vi "testFIFO.vi"() -> ()   [LabVIEW 2019]
panel:
  out "output array":dbl[](array[numeric])
  in  "Stop 2":bool
  out "average":dbl
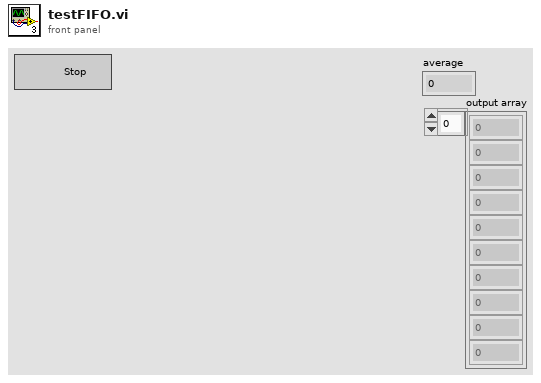
[diagram p1: front panel]
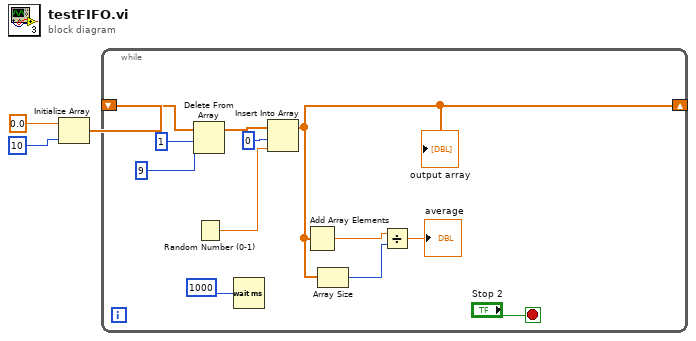
[diagram p0: block diagram]
diagram:
  n1 = Initialize Array(0.0 ("element"), 10 ("dimension size")) -> (w1:dbl[])
  n2 = while {
    shift-right: [w6] -> _
    shift-left: w1 -> [w13]
    stop <- "Stop 2" stop-if-true
    n3 = Delete From Array(array=w13, length=1, index=9) -> (array with subset deleted=w10:dbl[])  [unwired: 1 out]
    n4 = Random Number (0-1)() -> (number: 0 to 1=w15:dbl)
    n5 = Wait (ms)(milliseconds to wait=u32 1000) -> ()  [unwired: 1 out]
    n6 = Insert Into Array(array=w10, index=0, new element=w15) -> (w6:dbl[])
    "output array" <- w6
    n7 = Add Array Elements(numeric array=w6) -> (sum=w9:dbl)
    n8 = Array Size(array=w6) -> (size(s)=w8:i32)
    n9 = Divide(x=w9, y=w8) -> (x/y=→"average":dbl)
  }
